vi "Flatten modbus object to byte array1.vi"(11 "object":cluster{"object ID":u8, "value":string} {"object ID" format="%x"}) -> (3 "byte array":u8[](array[numeric]))   [LabVIEW 2021, in "NI_modbus_upd.lvlib" / "Standard Data Model1.lvclass"]
uses:
  Standard Data Model1.lvclass
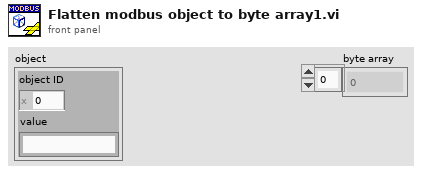
[diagram p1: front panel]
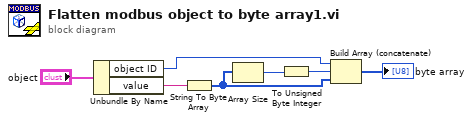
[diagram p0: block diagram]
diagram:
  n1 = Unbundle By Name("object") -> ("object ID"=w5:u8, "value"=w2:string)
  n2 = String To Byte Array(string=w2) -> (unsigned byte array=w4:u8[])
  n3 = Array Size(array=w4) -> (size(s)=w3:i32)
  n4 = To Unsigned Byte Integer(number=w3) -> (unsigned 8bit integer=w6:u8)
  n5 = Build Array (concatenate)(w5, w6, w4) -> (→"byte array":u8[])
